vi "buildLogEntry.vi"(8 "error in (no error)":errorcluster, 10 "command line":string, 11 "standard output":string) -> (0 "error out":errorcluster, 3 "String":string)   [LabVIEW 2013]
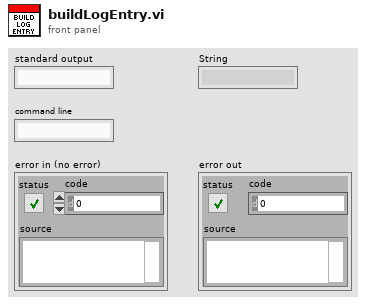
[diagram p1: front panel]
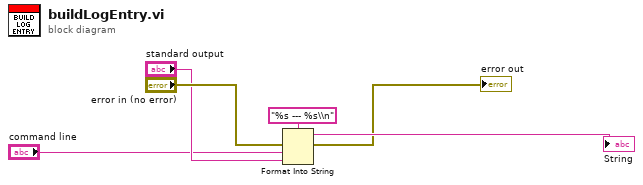
[diagram p0: block diagram]
diagram:
  n1 = Format Into String(format string="%s --- %s\\n", error in="error in (no error)", "command line", "standard output") -> (resulting string=→"String":string, error out=→"error out":errorcluster)  [unwired: 1 in]
